vi "LINX - Digital Read N Channels.vi"() -> ()   [LabVIEW 2014]
doc: "This example demonstrates how to read N channels of digital input from a LINX device."
uses:
  <vilib>/MakerHub/LINX/Public/Peripherals/Digital/Digital Read N Chans.vi
  <vilib>/MakerHub/LINX/Private/Local IO/LinxDigitalRead.vi
  <vilib>/MakerHub/LINX/Public/Utilities/Check Channel.vi
  <vilib>/MakerHub/LINX/Private/Local IO/Handle Errors.vi
  <vilib>/MakerHub/LINX/Public/Utilities/Open Local.vi
  <vilib>/MakerHub/LINX/Private/Utilties/Generate Error.vi
  Communication Channel.lvclass
  <vilib>/MakerHub/LINX/LMH-LINX.lvlib
  <vilib>/httpClient/LabVIEWHTTPClient.lvlib
panel:
  out "Values":bool[](array[boolean])
  out "Waveform Chart 9":dbl(graph)
  out "Waveform Chart 8":dbl(graph)
  out "Waveform Chart 7":dbl(graph)
  out "Bedroom":dbl(graph)
  out "Waveform Chart 5":dbl(graph)
  out "Waveform Chart 4":dbl(graph)
  out "Patio Door":dbl(graph)
  out "Backdoor and Living Room":dbl(graph)
  out "Waveform Chart":dbl(graph)
  out "Voltages":dbl[](array[numeric])
  out "Front Door":dbl(graph)
  in  "DI Channels":u8[](array[numeric])=[0, 1, 2, 3, 4, 5, 6]
  in  "Stop Button":bool
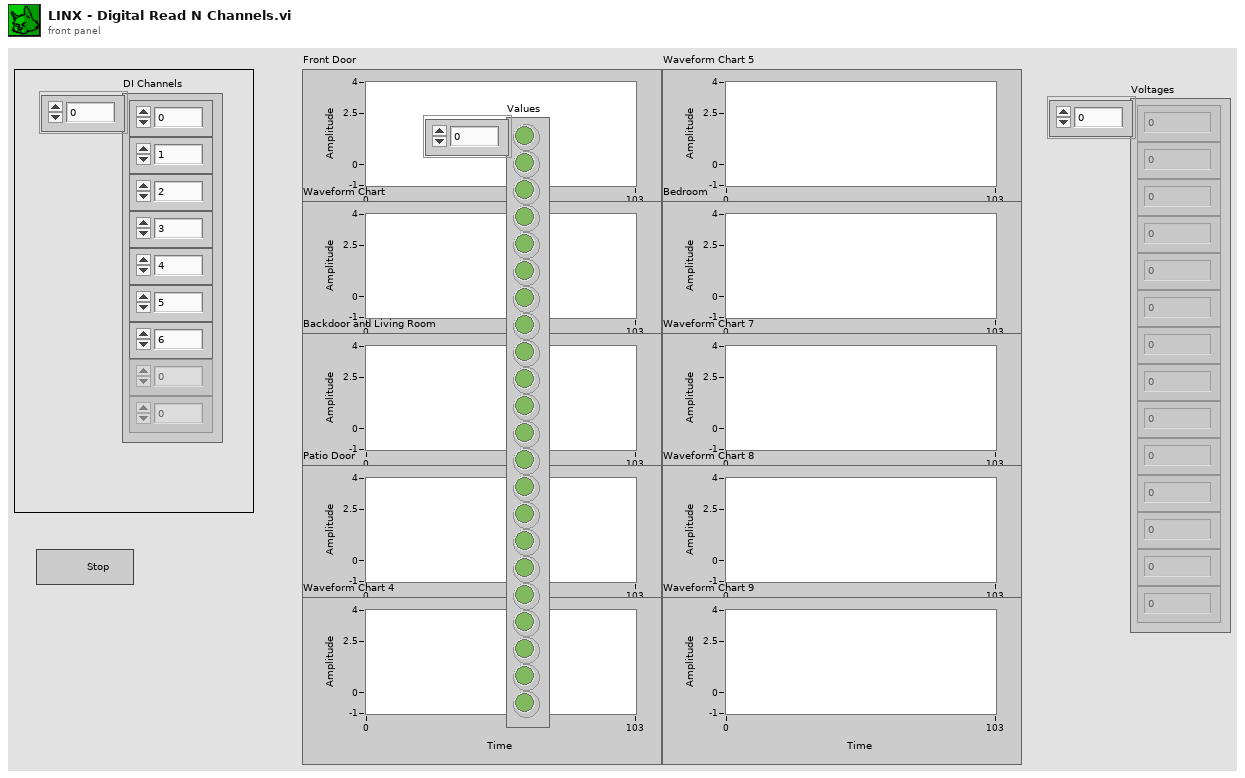
[diagram p1: front panel]
types:
  T1 = typedef "LMH-LINX.lvlib/LINX Ref.ctl" = cluster{"IO":T2, "Interface":T3, "LINX Device Config":T4}
  T2 = typedef "LMH-LINX.lvlib/Platform.ctl" = enum16{"Remote", "Local"}
  T3 = typedef "LMH-LINX.lvlib/Interface.ctl" = enum16{"Serial", "TCP"}
  T4 = typedef "LMH-LINX.lvlib/Device.lvlib/LINX Device Config.ctl" = cluster{"Interface":T3, "COM Port":refnum<visa-resource-name>, "TCP Configuration":T5, "Device Family":u8, "Device ID":u8, "Device Name":string, "TCP Ref":refnum<k5>, "Channels":T6}
  T5 = typedef "LMH-LINX.lvlib/Device.lvlib/TCP Config.ctl" = cluster{"IP Address":string, "Port":u16}
  T6 = typedef "LMH-LINX.lvlib/Channels.ctl" = cluster{"DI":u8[], "DO":u8[], "AI":u8[], "AO":u8[], "PWM":u8[], "QE":u8[], "UART":u8[], "I2C 2":u8[], "SPI":u8[], "CAN":u8[], "Servo":u8[], "AI Ref (V)":dbl, "AI Resolution (Bits)":u8, "AO Ref (V)":dbl, "AO Resolution (Bits)":u8}
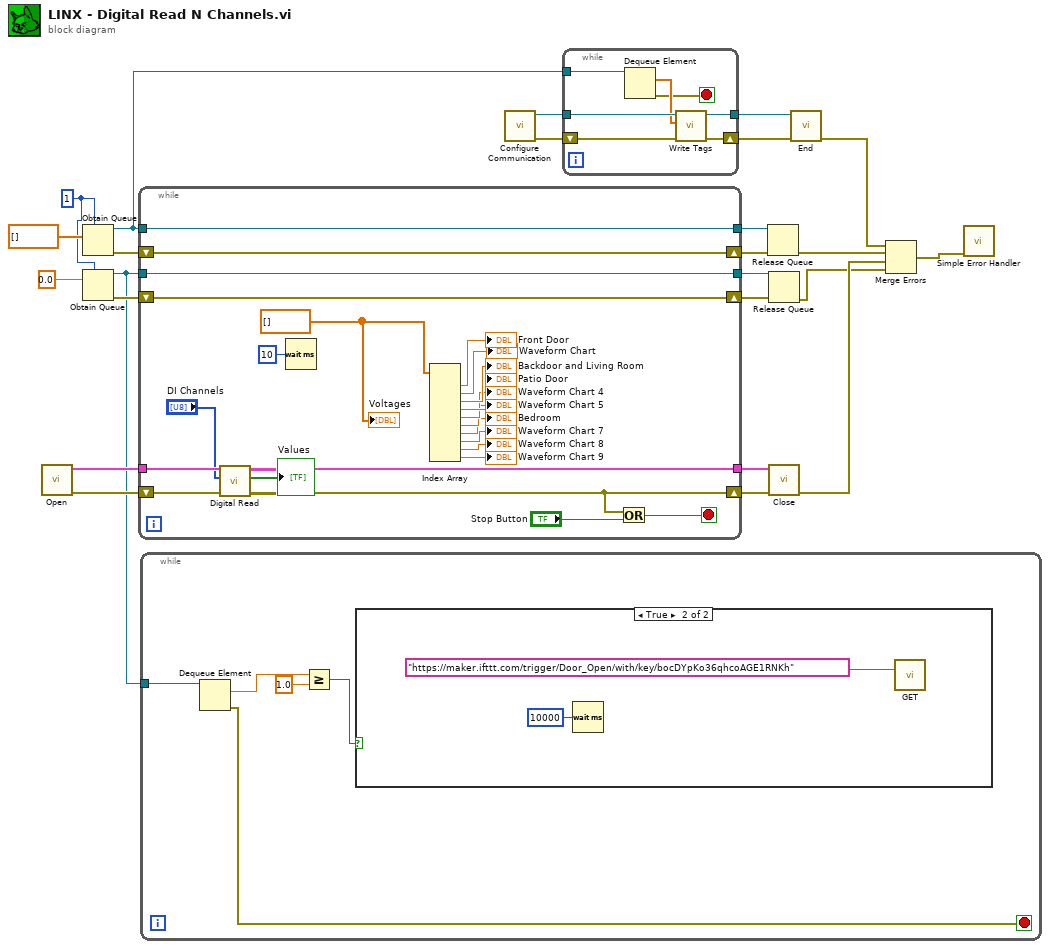
[diagram p0: block diagram]
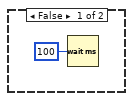
[diagram p2: hidden frame]
diagram:
  w1 = 1 ("max queue size (-1, unlimited)")
  n1 = call-poly <vilib>:"Open.vi"() -> ("Error Out"=w24:errorcluster, "LINX Resource"=w19:T1)  [unwired: 9 in, 1 out]
  n2 = Obtain Queue(max queue size (-1, unlimited)=w1, element data type=dbl[] [] ("Voltages")) -> (queue out=w16:refnum<queue>, error out=w11:errorcluster)  [unwired: 3 in, 1 out]
  n3 = Obtain Queue(max queue size (-1, unlimited)=w1, element data type=0.0 ("Numeric Control")) -> (queue out=w3:refnum<queue>, error out=w5:errorcluster)  [unwired: 3 in, 1 out]
  n4 = while {
    tunnel: [w28] -> w23
    shift-right: [w27] -> w22
    shift-left: w24 -> [w30]
    tunnel: w19 -> [w31]
    tunnel: w16 -> [w37]
    tunnel: [w37] -> w17
    shift-right: [w36] -> w10
    shift-left: w11 -> [w36]
    tunnel: w3 -> [w35]
    shift-right: [w33] -> w6
    shift-left: w5 -> [w33]
    tunnel: [w35] -> w2
    stop <- w39 stop-if-true
    w26 = dbl[] [] ("Voltages")
    n5 = call-poly <vilib>:"Digital Read.vi"("Error In"=w30, "DI Channels"="DI Channels", "LINX Resource"=w31) -> ("Error Out"=w27:errorcluster, "Values"=→"Values":bool[], "LINX Resource"=w28:T1)  [unwired: 6 in]
    n6 = Wait (ms)(milliseconds to wait=u32 10) -> ()  [unwired: 1 out]
    n7 = Index Array(array=w26) -> (element #1=→"Front Door":dbl, element #2=→"Waveform Chart":dbl, element #3=→"Backdoor and Living Room":dbl, element #4=→"Patio Door":dbl, element #5=→"Waveform Chart 4":dbl, element #6=→"Waveform Chart 5":dbl, element #7=→"Bedroom":dbl, element #8=→"Waveform Chart 7":dbl, element #9=→"Waveform Chart 8":dbl, element #10=→"Waveform Chart 9":dbl)  [unwired: 10 in]
    n8 = Or(x=w27, y="Stop Button") -> (x .or. y?=w39:bool)
    "Voltages" <- w26
  }
  n9 = while {
    tunnel: w3 -> [w53]
    stop <- w52 stop-if-true
    n10 = Dequeue Element(queue=w53) -> (element=w49:dbl, error out=w52:errorcluster)  [unwired: 2 in, 2 out]
    n11 = Greater Or Equal?(x=w49, y=1.0) -> (x >= y?=w50:bool)
    n12 = case shown="True" w50 {
      frame False {
        n13 = Wait (ms)(milliseconds to wait=u32 100) -> ()  [unwired: 1 out]
      }
      frame True {
        n14 = Wait (ms)(milliseconds to wait=u32 10000) -> ()  [unwired: 1 out]
        n15 = call <vilib>:"GET.vi"("url"="https://maker.ifttt.com/trigger/Door_Open/with/key/bocDYpKo36qhcoAGE1RNKh") -> ()  [unwired: 11 in, 4 out]
      }
    }
  }
  n16 = call "Configure Communication.vi"() -> ("error out"=w14:errorcluster, "Communication Channel.lvclass"=w15:refnum<class "Communication Channel.lvclass">)  [unwired: 10 in]
  n17 = while {
    tunnel: w16 -> [w63]
    tunnel: w15 -> [w62]
    shift-right: [w59] -> w13
    shift-left: w14 -> [w61]
    tunnel: [w57] -> w12
    stop <- w58 stop-if-true
    n18 = Dequeue Element(queue=w63) -> (element=w60:dbl[], error out=w58:errorcluster)  [unwired: 2 in, 2 out]
    n19 = call-dynamic "Write Tags.vi"("error in (no error)"=w61, "Array of Values"=w60, "Communication Channel in"=w62) -> ("error out"=w59:errorcluster, "Communication Channel out"=w57:refnum<class "Communication Channel.lvclass">)  [unwired: 7 in]
  }
  n20 = Release Queue(queue=w17, error in (no error)=w10) -> (error out=w8:errorcluster)  [unwired: 1 in, 2 out]
  n21 = Release Queue(queue=w2, error in (no error)=w6) -> (error out=w4:errorcluster)  [unwired: 1 in, 2 out]
  n22 = call <vilib>:"Close.vi"("Error In"=w22, "LINX Resource"=w23) -> ("Error Out"=w9:errorcluster)  [unwired: 9 in]
  n23 = call-dynamic "End.vi"("error in (no error)"=w13, "Communication Channel in"=w12) -> ("error out"=w20:errorcluster)  [unwired: 8 in, 1 out]
  n24 = Merge Errors(w20, w8, w9, w4) -> (w21:errorcluster)
  n25 = call <vilib>:"Simple Error Handler.vi"("error in (no error)"=w21) -> ()  [unwired: 4 in, 5 out]
